vi "Force Simulation.vi"() -> ()   [LabVIEW 2015]
uses:
  <vilib>/Simulation/Scripting/Companion Diagram/SimConfigNode/SimParams.ctl
  <vilib>/Simulation/Scripting/Companion Diagram/SimConfigNode/_simSolvers.ctl
  <vilib>/Simulation/Implementation/Shared/SIMSCR Execution Mode.ctl
  <vilib>/Platform/TimedLoop/XDataNode/timing_clust.ctl
  <vilib>/Platform/TimedLoop/XDataNode/nitl_modes.ctl
  <vilib>/Platform/TimedLoop/XDataNode/wakeup.ctl
  <vilib>/Simulation/Param Hierarchy/Typedefs/SIMPH Param Control Actions.ctl
  <vilib>/Simulation/Implementation/Shared/SIM limit type.ctl
  <vilib>/Simulation/Implementation/Shared/NILVSim_ParamChanged.vi
  <vilib>/Simulation/Implementation/Shared/NILVSim_FinishedLate.vi
  <vilib>/Simulation/Implementation/Shared/NILVSIM_BeginStep.vi
  <vilib>/Simulation/DataSources/Implementation/NILVSim Step.llb/SIM Step (scalar).vi
  <vilib>/Simulation/ContinuousLinear/Implementation/NILVSim Transfer Function.llb/SIM Transfer Function Distributor (SISO CD).vi
  <vilib>/Simulation/ContinuousLinear/Implementation/NILVSim Transfer Function.llb/SIM Transfer Function Collector (SISO).vi
  <vilib>/Simulation/ContinuousLinear/Implementation/NILVSim Integrator new.llb/SIM Integrator distributor (scalar).vi
  <vilib>/Simulation/SignalArithmetic/Implementation/NILVSim Gain.llb/SIM Gain (scalar).vi
  <vilib>/Simulation/ContinuousLinear/Implementation/NILVSim Derivative.llb/SIM derivative (scalar).vi
  <vilib>/Simulation/ContinuousLinear/Implementation/NILVSim Integrator new.llb/SIM Integrator collector (scalar).vi
  <vilib>/Simulation/Nonlinear/Implementation/NILVSim Saturation.llb/SIM Saturation (scalar).vi
  <vilib>/Simulation/SignalDisplay/Implementation/NILVSim Time Waveform.llb/SIM Time Waveform (vector).vi
  <vilib>/Simulation/Implementation/Shared/NILVSim_Manager.vi
  <vilib>/Utility/error.llb/Clear Errors.vi
  <vilib>/Simulation/Implementation/Shared/NILVSim_FinalizeModel.vi
  <vilib>/Simulation/Implementation/Shared/SIM Unbundle Sim Info.vi
  <vilib>/Simulation/Implementation/Shared/SIMSH Read Queue.vi
  <vilib>/Simulation/Implementation/Shared/NILVSim_Initialize.vi
  <vilib>/addons/Control Design/_Model Construction/Model Creation.llb/CD Construct Transfer Function Model.vi
  <vilib>/addons/Control Design/_Model Construction/Model Creation.llb/Model Creation SubVI/cd_Create Transfer Function Model.vi
  <vilib>/Simulation/Utility/Implementation/NILVSim Get Time and IsAcceptedStep.vi
  <vilib>/Simulation/Implementation/Shared/NILVSim_GetModelError.vi
  <vilib>/Simulation/Implementation/Shared/SIM Bundle Sim Info.vi
  <vilib>/addons/Control Design/_Utility/Model Viewer.llb/Model Viewer SubVI/cd_Draw Transfer Function Equation (TF).vi
  <vilib>/addons/Control Design/_Time Response Analysis/Time Response.llb/Time Response subVI/cd_Step Response (Transfer Function).vi
  <vilib>/addons/Control Design/_Frequency Response Analysis/Frequency Response.llb/Frequency Response subVI/cd_Bode (Transfer Function).vi
  <vilib>/Simulation/Scripting/Companion Diagram/SimConfigNode/SimDog.xnode
  <vilib>/addons/Control Design/_Model Construction/Model Typedefs.llb/CD Transfer Function Model (MIMO).ctl
  <vilib>/addons/Control Design/_Model Construction/Model Typedefs.llb/CD General Elements.ctl
  <vilib>/addons/Control Design/_Model Construction/Model Typedefs.llb/CD Transfer Function Model (SISO).ctl
  <vilib>/Platform/TimedLoop/XDataNode/XDataNode.xnode
  <vilib>/Simulation/Implementation/XNodeFramework/SimXNode/SimX.xnode
  <vilib>/Simulation/ContinuousLinear/Implementation/NILVSim Integrator new.llb/SIM Integrator (scalar).vi
  <vilib>/addons/Control Design/_Frequency Response Analysis/NI_CD_Frequency Response.lvlib
  <vilib>/addons/Control Design/_Time Response Analysis/NI_CD_Time Response.lvlib
  <vilib>/addons/Control Design/_Utility/NI_CD_Model Viewer.lvlib
  <vilib>/addons/Control Design/_Model Construction/NI_LinSys_Model Typedefs.lvlib
  <vilib>/Simulation/ContinuousLinear/Implementation/NILVSim Transfer Function.llb/SIM Transfer Function (SISO CD).vi
  <vilib>/addons/Control Design/_Model Construction/NI_LinSys_Model Creation.lvlib
  <vilib>/Platform/TimedLoop/XDataNode/XDNodeRunTimeDep.lvlib
  <vilib>/Simulation/Implementation/Shared/NI_SIM_Implementation.lvlib
panel:
  in  "Rm":dbl format="%#_13g"
  in  "Desired Force (N)":dbl format="%#_13g"
  out "Simulated Data":dbl(graph)
  out "Step Response Graph":cluster{"time":dbl[], dbl[]}[](graph)
  out "Bode Phase":cluster{"W":dbl[], "Magnitude":dbl[]}[](graph)
  out "Bode Magnitude":cluster{"W":dbl[], "Magnitude":dbl[]}[](graph)
  out "2D Picture of Equation":picture
  out "Current Value VS Desired Value":waveform(dbl)[](graph)
  out "Voltage VS Time":T1(graph)
  in  "Kd":dbl
  in  "Ki":dbl
  out "Error VS Time":cluster{"Constant":dbl, "Result":dbl}(graph)
  in  "Kp":dbl
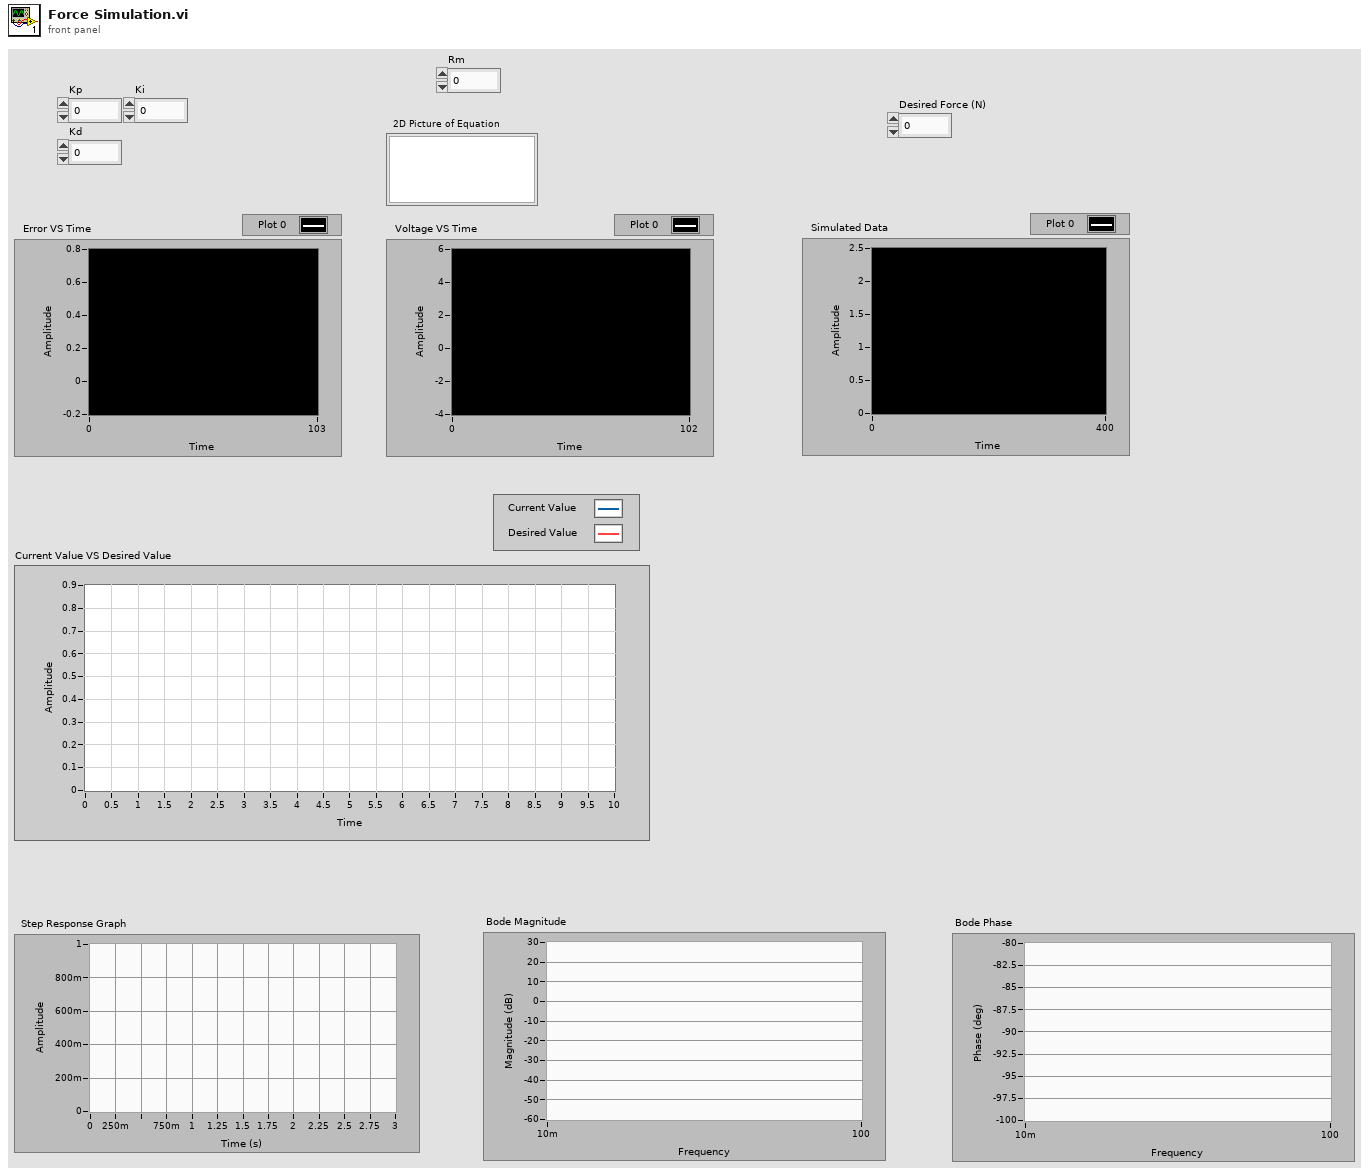
[diagram p1: front panel]
types:
  T1 = cluster{"output":dbl, "Constant 5":dbl, "Constant 2":dbl}
  T2 = typedef "NI_LinSys_Model Typedefs.lvlib/CD Transfer Function Model (MIMO).ctl" = cluster{"properties":T3, "transfer function(s)":T4[][]}
  T3 = typedef "NI_LinSys_Model Typedefs.lvlib/CD General Elements.ctl" = cluster{"Model name":string, "Input names":string[], "Output names":string[], "Input Delays":dbl[], "Output Delays":dbl[], "Sampling Time":dbl, "Notes":string}
  T4 = typedef "NI_LinSys_Model Typedefs.lvlib/CD Transfer Function Model (SISO).ctl" = cluster{"Numerator":dbl[], "Denominator":dbl[], "delay":dbl}
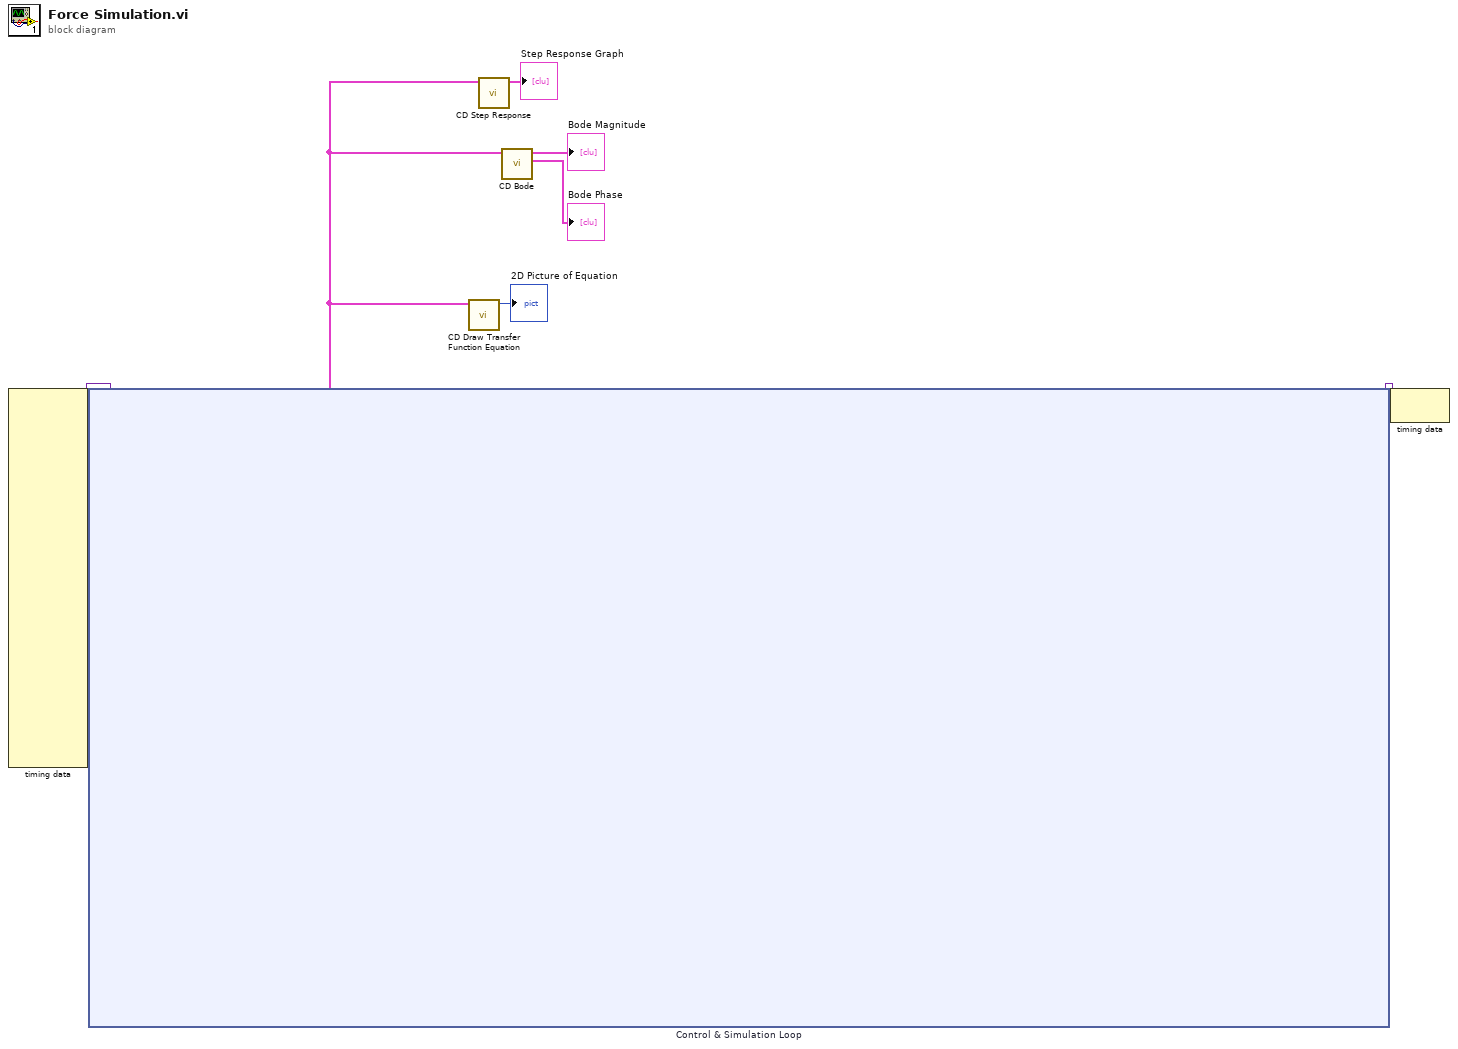
[diagram p0: block diagram]
diagram:
  n1 = node-c288() -> (w7:variant)  [unwired: 24 in]
  n2 = node-c254 "Control & Simulation Loop"(w7) -> (w6:variant, w1:T2)
  n3 = call-poly <vilib>:"CD Draw Transfer Function Equation.vi"("Transfer Function Model"=w1) -> ("Equation"=→"2D Picture of Equation":picture)  [unwired: 8 in, 2 out]
  n4 = call-poly <vilib>:"CD Step Response.vi"("Transfer Function Model"=w1) -> ("Step Response Graph"=→"Step Response Graph":cluster{"time":dbl[], dbl[]}[])  [unwired: 8 in, 2 out]
  n5 = call-poly <vilib>:"CD Bode.vi"("Transfer Function Model"=w1) -> ("Bode Phase"=→"Bode Phase":cluster{"W":dbl[], "Magnitude":dbl[]}[], "Bode Magnitude"=→"Bode Magnitude":cluster{"W":dbl[], "Magnitude":dbl[]}[])  [unwired: 6 in, 3 out]
  n6 = node-c288(w6) -> ()  [unwired: 1 out]
